vi "Preview Next Message.vi"(0 "message queue in":T3, 1 "ignore error on termination message (F)":bool, 7 "termination list ([Exit])":string[](array[string])=["Exit"], 9 "timeout (1 ms)":i32=1, 11 "error in":errorcluster) -> (3 "termination message?":bool, 4 "message queue out":T3, 6 "message name":string, 8 "message value":string, 10 "timed out?":bool, 13 "acknowledge":bool, 14 "message":T1, 15 "error out":errorcluster)   [LabVIEW 2015, in "Car Wash.lvlib" / "AMC.lvlib"]
doc: "Previews the next message from the message queue passed in, but does not remove it from the queue. If the returned message matches any of the message names listed in \"termination list\" the \"termination message?\" indicator will return True."
uses:
  AMC.lvlib
  Globals.vi
  Message.ctl
  Message Queue.ctl
  Tools/Keyed Array/KeyedArray.ctl
  Tools/Keyed Array/Tools_KeyedArray.lvlib
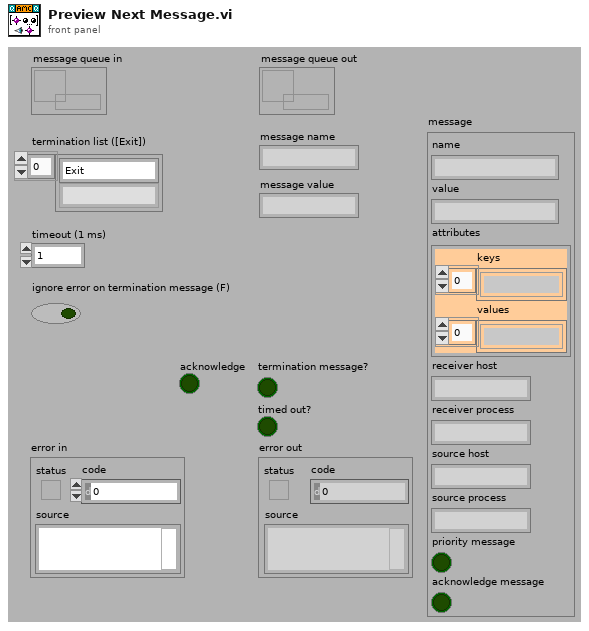
[diagram p1: front panel]
types:
  T1 = typedef "Car Wash.lvlib/AMC.lvlib/Message.ctl" = cluster{"name":string, "value":string, "attributes":T2, "receiver host":string, "receiver process":string, "source host":string, "source process":string, "priority message":bool, "acknowledge message":bool}
  T2 = typedef "Car Wash.lvlib/Tools_KeyedArray.lvlib/KeyedArray.ctl" = cluster{"keys":string[], "values":string[]}
  T3 = typedef "Car Wash.lvlib/AMC.lvlib/Message Queue.ctl" = refnum<queue>
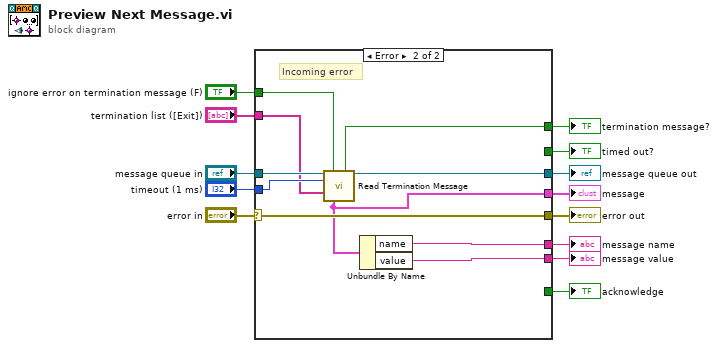
[diagram p0: block diagram]
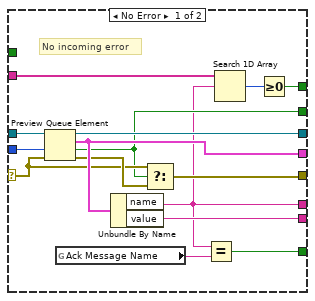
[diagram p2: hidden frame]
diagram:
  n1 = case shown="Error" "error in" {
    selector: "error in" -> [w18 w38]
    tunnel: "message queue in" -> [w28 w37]
    tunnel: [w27 w32] -> w11
    tunnel: [w15 w30] -> w13
    tunnel: "timeout (1 ms)" -> [w26 w36]
    tunnel: [w19 w38] -> w12
    tunnel: [w24 w29] -> w10
    tunnel: [w25 w31] -> w9
    tunnel: "termination list ([Exit])" -> [w23 w33]
    tunnel: [w21 w34] -> w8
    tunnel: "ignore error on termination message (F)" -> [_ w35]
    tunnel: [w17 _] -> w2
    tunnel: [w14 _] -> w1
    frame No Error {
      # "No incoming error"
      n2 = Preview Queue Element(queue=w28, timeout in ms (-1)=w26, error in (no error)=w18) -> (queue out=w27:T3, element=w25:T1, timed out?=w17:bool, error out=w20:errorcluster)
      n3 = global read "Globals.vi" "Ack Message Name"() -> (w16:string)
      n4 = Unbundle By Name(w25) -> ("name"=w15:string, "value"=w24:string)
      n5 = Select(t=w18, s=w17, f=w20) -> (s? t:f=w19:errorcluster)
      n6 = Equal?(x=w15, y=w16) -> (x = y?=w14:bool)
      n7 = Search 1D Array(1D array=w23, element=w15) -> (index of element=w22:i32)  [unwired: 1 out]
      n8 = Greater Or Equal To 0?(x=w22) -> (x >= 0?=w21:bool)
    }
    frame Error {
      # "Incoming error"
      n9 = call "Read Termination Message.vi"("message queue in"=w37, "ignore error on termination message (F)"=w35, "timeout (1 ms)"=w36, "termination list ([Exit])"=w33) -> ("termination message"=w34:bool, "message queue out"=w32:T3, "message"=w31:T1)  [unwired: 9 in]
      n10 = Unbundle By Name(w31) -> ("name"=w30:string, "value"=w29:string)
    }
  }
  "message queue out" <- w11
  "message name" <- w13
  "error out" <- w12
  "message value" <- w10
  "message" <- w9
  "termination message?" <- w8
  "timed out?" <- w2
  "acknowledge" <- w1
